vi "DereferencingPointerToArrayOfSimpleStructUsingGetValueByPointer.vi"(8 "error in (no error)":errorcluster, 10 "Length":i32, 11 "Address (Pointer)":i64) -> (0 "error out":errorcluster, 3 "Destination":T1[](array[typedef]))   [LabVIEW 2009, in "LabVIEWWrapper_PassingDataSampleDLL.lvlib"]
uses:
  LabVIEWWrapper_PassingDataSampleDLL.lvlib
  CustomControlsForStructs/SimpleStruct Circle.ctl
  <vilib>/Utility/importsl/GetValueByPointer/GetValueByPointer.xnode
  <vilib>/Utility/importsl/GetValueByPointer/datatype.ctl
  Program Files (x86)/National Instruments/LabVIEW 2009/resource/lvimptsl.dll
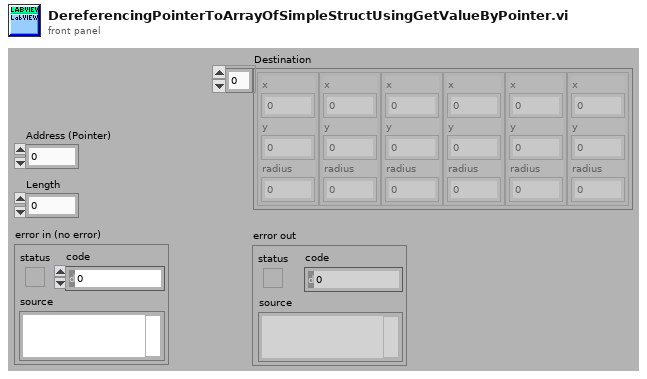
[diagram p1: front panel]
types:
  T1 = typedef "LabVIEWWrapper_PassingDataSampleDLL.lvlib/SimpleStruct Circle.ctl" = cluster{"x":sgl, "y":sgl, "radius":sgl}
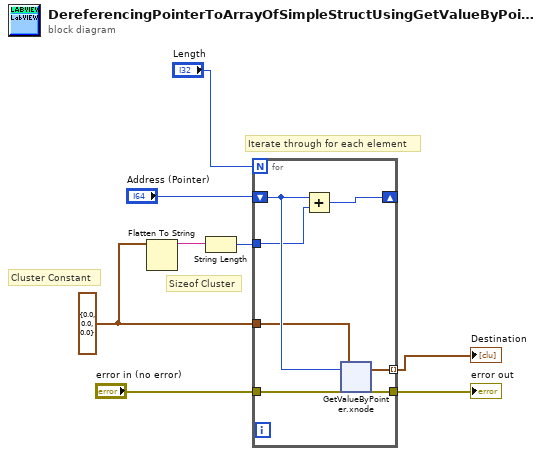
[diagram p0: block diagram]
diagram:
  w2 = cluster{"x":sgl, "y":sgl, "radius":sgl} {"x"=0.0, "y"=0.0, "radius"=0.0} ("Circle")
  # "Sizeof Cluster"
  # "Iterate through for each element"
  # "Cluster Constant"
  n1 = Flatten To String(anything=w2) -> (data string=w5:string)  [unwired: 3 in, 2 out]
  n2 = String Length(string=w5) -> (length=w3:i32)
  n3 = for {
    N: "Length" -> [_]
    shift-right: [w15] -> _
    shift-left: "Address (Pointer)" -> [w14]
    tunnel: [w13] -> w1 mode=indexing
    tunnel: [w12] -> w6
    tunnel: "error in (no error)" -> [w11]
    tunnel: w3 -> [w10]
    tunnel: w2 -> [w9]
    n4 = Add(x=w14, y=w10) -> (x+y=w15:i64)
    n5 = xnode "GetValueByPointer.xnode"("Pointer"=w14, "InputType"=w9, "ErrorIn"=w11) -> ("Output"=w13:cluster{"x":sgl, "y":sgl, "radius":sgl}, "ErrorOut"=w12:errorcluster)  [unwired: 1 in]
  }
  "error out" <- w6
  "Destination" <- w1
